vi "LeerCorriente.vi"(0 "output cluster":T1, 1 "Boolean":bool) -> (2 "error out":errorcluster, 3 "data":dbl, 4 "Cluster":T1, 5 "Boolean 2":bool)   [LabVIEW 2017]
uses:
  <vilib>/DAQmx/read.llb/DAQmx Read (Analog 1D DBL 1Chan NSamp).vi
  <vilib>/DAQmx/miscellaneous.llb/DAQmx Fill In Error Info.vi
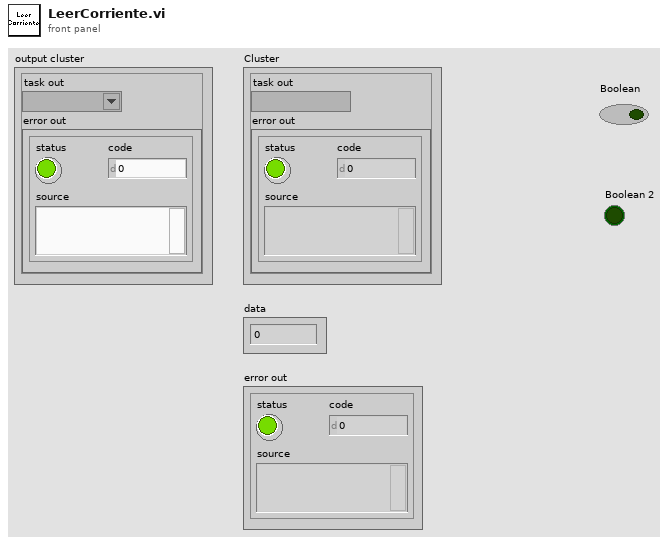
[diagram p1: front panel]
types:
  T1 = cluster{"task out":refnum<k21>, "error out":errorcluster}
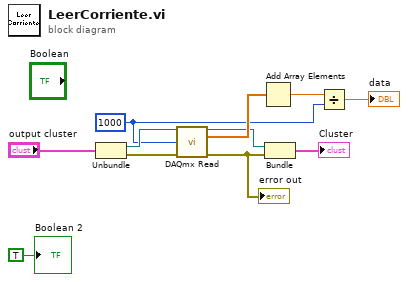
[diagram p0: block diagram]
diagram:
  w1 = 1000
  n1 = Unbundle("output cluster") -> ("task out"=w3:refnum<k21>, "error out"=w4:errorcluster)
  n2 = call-poly <vilib>:"DAQmx Read.vi"("task/channels in"=w3, "number of samples per channel"=w1, "error in"=w4) -> ("task out"=w5:refnum<k21>, "data"=w8:dbl[], "error out"=w2:errorcluster)  [unwired: 10 in]
  "error out" <- w2
  n3 = Add Array Elements(numeric array=w8) -> (sum=w7:dbl)
  n4 = Bundle("task out"=w5, "error out"=w2) -> (→"Cluster":T1)  [unwired: 1 in]
  n5 = Divide(x=w7, y=w1) -> (x/y=→"data":dbl)
  "Boolean 2" <- TRUE
